vi "arraytrack.vi"(9 "freq":dbl, 10 "samples":cdb[](array[numeric]), 11 "samples num":u32) -> (0 "error out":errorcluster, 1 "max":dbl, 2 "spectrum":cluster{dbl[], dbl[]}(graph))   [LabVIEW 2020]
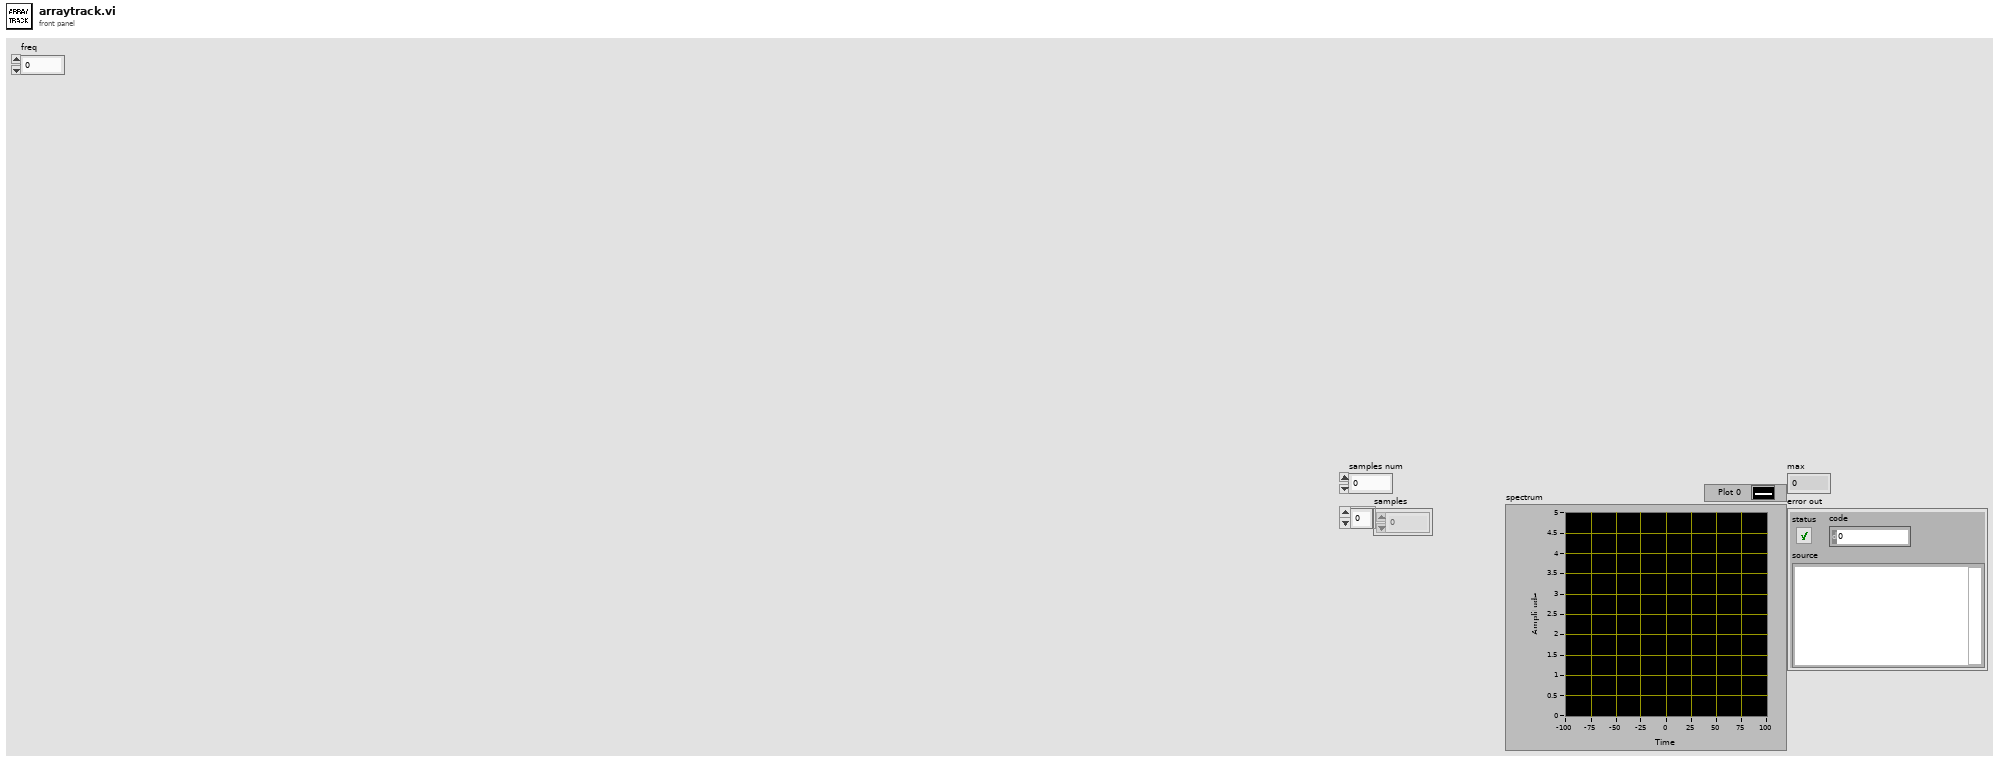
[diagram p1: front panel]
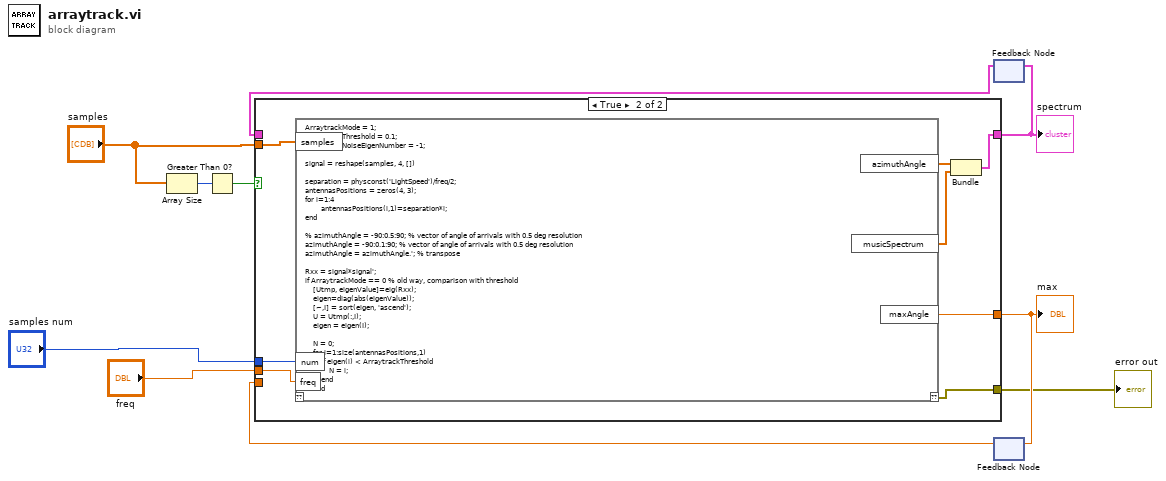
[diagram p0: block diagram]
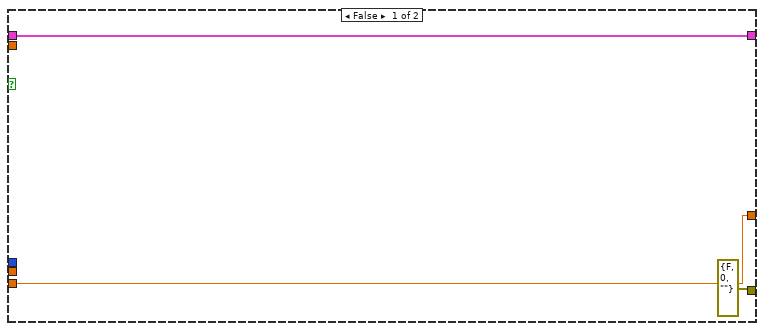
[diagram p2: hidden frame]
diagram:
  n1 = Array Size(array="samples") -> (size(s)=w4:i32)
  n2 = Greater Than 0?(x=w4) -> (x > 0?=w3:bool)
  n3 = feedback #1() -> (w9:cluster{dbl[], dbl[]})  [unwired: 1 in]
  n4 = feedback #2() -> (w7:dbl)  [unwired: 1 in]
  n5 = case shown="True" w3 {
    tunnel: "freq" -> [_ w21]
    tunnel: [w13 w18] -> w10
    tunnel: w9 -> [w13 _]
    tunnel: [w12 w17] -> w8
    tunnel: w7 -> [w12 _]
    tunnel: "samples" -> [_ w16]
    tunnel: "samples num" -> [_ w15]
    tunnel: [errorcluster {"status"=FALSE, "code"=0, "source"=""} ("error IO") w14] -> w1
    frame False {
    }
    frame True {
      n6 = script code="ArraytrackMode = 1;\nArraytrackThreshold = 0.1;\nArraytrackNoiseEigenNumber = -1;\n\nsignal = reshape(samples, 4, [])\n\nseparation = physconst('LightSpeed')/freq/2;\nantennasPositions = zeros(4, 3);\nfor i=1:4\n        antennasPositions(i,1)=separation*i;\nend\n\n% azimuthAngle = -90:0.5:90; % vector of angle of arrivals with 0.5 deg resolution\nazimuthAngle = -90:0.1:90; % vector of angle of arrivals with 0.5 deg resolution\nazimuthAngle = azimuthAngle.'; % transpose\n\nRxx = signal*signal';\nif ArraytrackMode == 0 % old way, comparison with threshold\n    [Utmp, eigenValue]=eig(Rxx);\n    eigen=diag(abs(eigenValue));\n    [~,I] = sort(eigen, 'ascend');\n    U = Utmp(:,I);\n    eigen = eigen(I);\n    \n    N = 0;\n    for i=1:size(antennasPositions,1)\n        if eigen(i) < ArraytrackThreshold\n            N = i;\n        end\n    end\n    \n    if N == 0\n        N = 1;\n    end\n    \n    En = U(:,1:N);\n    \n    if N == 0\n        error('Arraytrack: sources not found')\n    end\nelseif ArraytrackMode == 1\n    [Utmp,eigenValue] = eig(Rxx);\n    eigen=diag(abs(eigenValue));\n    [~,I] = sort(eigen, 'ascend');\n    U = Utmp(:,I);\n    eigen = eigen(I);\n    \n    N = ArraytrackNoiseEigenNumber;\n    if N < 0\n        N = length(eigen)+N;\n    end\n    En = U(:,1:N);\nend\n\nelevationAngle = zeros(size(azimuthAngle)); % vector of zeros with the same size as az\nsteeringVectors = steeringVectorsCreate(antennasPositions, [azimuthAngle + 90,elevationAngle], freq);\nmusicSpectrum=zeros(1,length(azimuthAngle));\nfor i=1:length(azimuthAngle)\n    musicSpectrum(i)=-10*log10(abs(steeringVectors(:,i)'*(En*En')*steeringVectors(:,i)));\nend\n%musicSpectrum = musicSpectrum.';\nmusicSpectrum = musicSpectrum - min(musicSpectrum);\n\n[~, ind] = max(musicSpectrum);\nif length(azimuthAngle) > 0\n    maxAngle = azimuthAngle(ind);\nend\n\nazimuthAngle = azimuthAngle.'; % transpose" ("Script Node")("samples"=w16, "num"=w15, "freq"=w21) -> ("??"=w14:errorcluster, "musicSpectrum"=w19:dbl[], "azimuthAngle"=w20:dbl[], "maxAngle"=w17:dbl)  [unwired: 1 in]
      n7 = Bundle(w20, w19) -> (w18:cluster{dbl[], dbl[]})  [unwired: 1 in]
    }
  }
  "spectrum" <- w10
  "max" <- w8
  "error out" <- w1
  n8 = feedback-in #1(w10) -> ()
  n9 = feedback-in #2(w8) -> ()
